vi "add channel to configuration.vi"(8 "error in":errorcluster, 10 "TBM channel in":refnum<class "TBM channel.lvclass">, 11 "TDMS datalogger configuration in":refnum<class "TDMS datalogger configuration.lvclass">) -> (0 "error out":errorcluster, 3 "TDMS datalogger configuration out":refnum<class "TDMS datalogger configuration.lvclass">)   [LabVIEW 2013, in "TDMS datalogger configuration.lvclass"]
uses:
  TDMS datalogger configuration.lvclass
  <vilib>/NI/Tag Bus Module Framework/channel/TBM channel.lvclass
  <vilib>/NI/Tag Bus/tag/tag descriptor.lvclass/tag descriptor.ctl
  TDMS datalogger configuration.lvclass/TDMS datalogger configuration.ctl
  Read channels.vi
  Write channels.vi
  <vilib>/NI/Tag Bus/tag/read tag name.vi
  <vilib>/NI/Tag Bus/tag/tag descriptor.lvclass
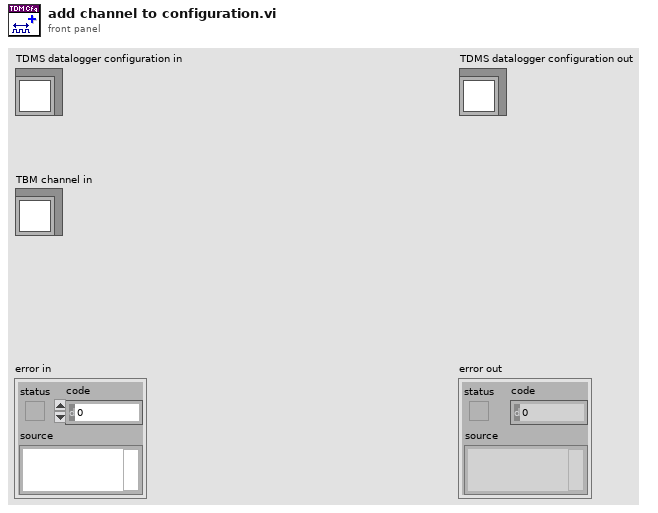
[diagram p1: front panel]
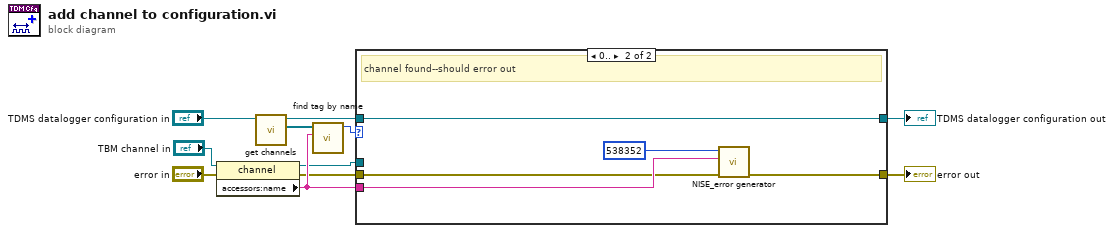
[diagram p0: block diagram]
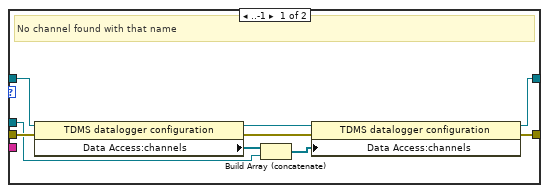
[diagram p2: hidden frame]
diagram:
  n1 = property class="channel"(reference="TBM channel in", error in="error in") -> (reference out=w7:refnum<class "TBM channel.lvclass">, error out=w6:errorcluster, "accessors:name"=w9:string)
  n2 = call-dynamic "get channels.vi"("module configuration in"="TDMS datalogger configuration in") -> ("channels"=w11:refnum<class "TBM channel.lvclass">[], "module configuration out"=w8:refnum<class "TDMS datalogger configuration.lvclass">)  [unwired: 9 in]
  n3 = call <vilib>:"find tag by name.vi"("name"=w9, "tags in"=w11) -> ("index"=w10:i32)  [unwired: 9 in]
  n4 = case shown="0.." w10 {
    tunnel: [w13 w25] -> w1
    tunnel: w9 -> [_ w23]
    tunnel: w6 -> [w20 w22]
    tunnel: w8 -> [w19 w21]
    tunnel: w7 -> [w14 _]
    tunnel: [w12 w21] -> w2
    frame ..-1 {
      # "No channel found with that name"
      n5 = property class="TDMS datalogger configuration"(reference=w19, error in=w20) -> (reference out=w18:refnum<class "TDMS datalogger configuration.lvclass">, error out=w17:errorcluster, "Data Access:channels"=w16:refnum<class "TBM channel.lvclass">[])
      n6 = Build Array (concatenate)(w16, w14) -> (w15:refnum<class "TBM channel.lvclass">[])
      n7 = property class="TDMS datalogger configuration"(reference=w18, error in=w17, "Data Access:channels"=w15) -> (reference out=w12:refnum<class "TDMS datalogger configuration.lvclass">, error out=w13:errorcluster)
    }
    frame 0.. {
      # "channel found--should error out"
      n8 = call <vilib>:"NISE_error generator.vi"("error in"=w22, "append error message"=w23, "error code (0)"=538352) -> ("error out"=w25:errorcluster)  [unwired: 6 in]
    }
  }
  "error out" <- w1
  "TDMS datalogger configuration out" <- w2
